vi "Configure Measurement Averaging.vi"(8 "error in (no error)":errorcluster, 9 "Enable Step Detection (T: Enable)":bool=TRUE, 10 "Voltage Average Value (0: 4)":i32(ring) items=["4", "8", "16", "32", "64", "128"], 11 "VISA resource name":refnum<visa-resource-name>) -> (0 "error out":errorcluster, 3 "VISA resource name out":refnum<visa-resource-name>)   [LabVIEW 2011, in "Agilent N432A.lvlib"]
doc: "Configures the voltage measurement averaging used in incident power calculation and sets the step detection."
uses:
  <instrlib>/Agilent N432A/Agilent N432A.lvlib
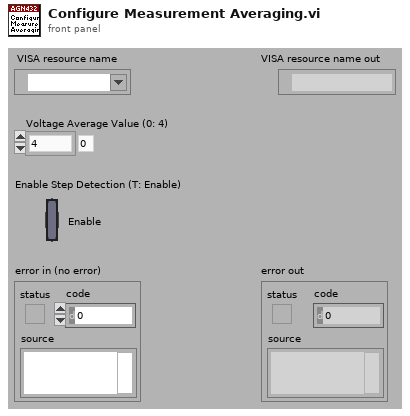
[diagram p1: front panel]
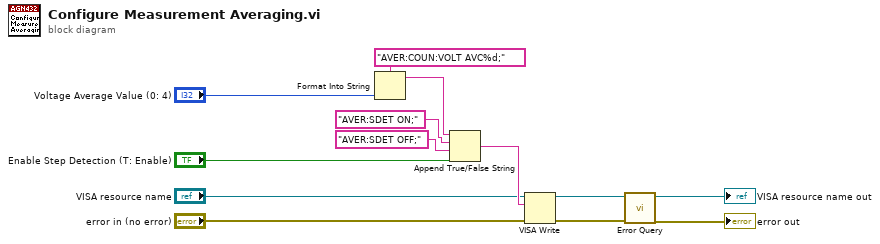
[diagram p0: block diagram]
diagram:
  n1 = Format Into String(format string="AVER:COUN:VOLT AVC%d;", "Voltage Average Value (0: 4)") -> (resulting string=w11:string)  [unwired: 2 in, 1 out]
  n2 = Append True/False String(1:"Enable Step Detection (T: Enable)", 2:"AVER:SDET OFF;", 3:"AVER:SDET ON;", 4:w11) -> (0:w7:string)
  n3 = VISA Write(VISA resource name="VISA resource name", write buffer=w7, error in (no error)="error in (no error)") -> (VISA resource name out=w4:refnum<visa-resource-name>, error out=w3:errorcluster)  [unwired: 1 out]
  n4 = call <instrlib>:"Error Query.vi"("error in (no error)"=w3, "VISA resource name"=w4) -> ("error out"=→"error out":errorcluster, "VISA resource name out"=→"VISA resource name out":refnum<visa-resource-name>)  [unwired: 6 in, 2 out]
